vi "Configure Trigger (Edge Then Edge - Setting).vi"(8 "error in (no error)":errorcluster, 9 "Delay Time (5E-7 seconds)":dbl=5e-07, 10 "Delay Trigger Count (1)":i32=1, 11 "VISA resource name":refnum<visa-resource-name>) -> (0 "error out":errorcluster, 3 "VISA resource name out":refnum<visa-resource-name>)   [LabVIEW 2023, in "Keysight-DSQx3014T.lvlib"]
doc: "Configures the settings of Delay(Edge Then Edge) trigger mode."
uses:
  Keysight-DSQx3014T.lvlib
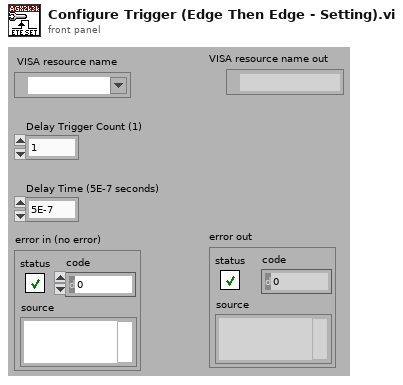
[diagram p1: front panel]
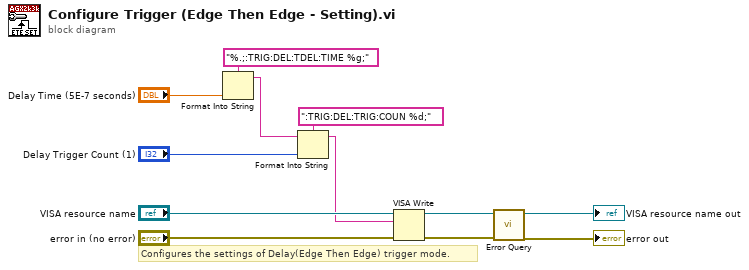
[diagram p0: block diagram]
diagram:
  # "Configures the settings of Delay(Edge Then Edge) trigger mode."
  n1 = Format Into String(format string="%.;:TRIG:DEL:TDEL:TIME %g;", "Delay Time (5E-7 seconds)") -> (resulting string=w10:string)  [unwired: 2 in, 1 out]
  n2 = Format Into String(format string=":TRIG:DEL:TRIG:COUN %d;", initial string=w10, "Delay Trigger Count (1)") -> (resulting string=w1:string)  [unwired: 1 in, 1 out]
  n3 = VISA Write(VISA resource name="VISA resource name", write buffer=w1, error in (no error)="error in (no error)") -> (VISA resource name out=w5:refnum<visa-resource-name>, error out=w4:errorcluster)  [unwired: 1 out]
  n4 = call "Error Query.vi"("error in (no error)"=w4, "VISA resource name"=w5) -> ("error out"=→"error out":errorcluster, "VISA resource name out"=→"VISA resource name out":refnum<visa-resource-name>)  [unwired: 8 out]
